vi "Read CSV.vi"(8 "error in (no error)":errorcluster caption="Error In", 10 "Source":string, 11 "Data Path":path=path "D:/NBT/01-Project/02-Processing/NBT-TestPlatform V2/NBT-TestPlatform V2.0.2/Config/NBT/NBT_V1.0.0/Project/0001_HZKD_ST01/00_DataSource/001_PLC/01_PLC/Data.xlsx") -> (0 "error out":errorcluster caption="Error Out", 1 "Data":T1(c390), 2 "Identifier List":T2[](array[typedef]), 3 "Identifiers Out":map{string, T2}(c390), 4 "Value Out":string[][](array[string]), 5 "Identifiers":string, 6 "Identifiers Out":string[](array[string]), 7 "Title":string[](array[string]))   [LabVIEW 2020]
uses:
  Global/Data Global/SDQ Data Type.ctl
  <vilib>/Utility/file.llb/Read Delimited Spreadsheet (string).vi
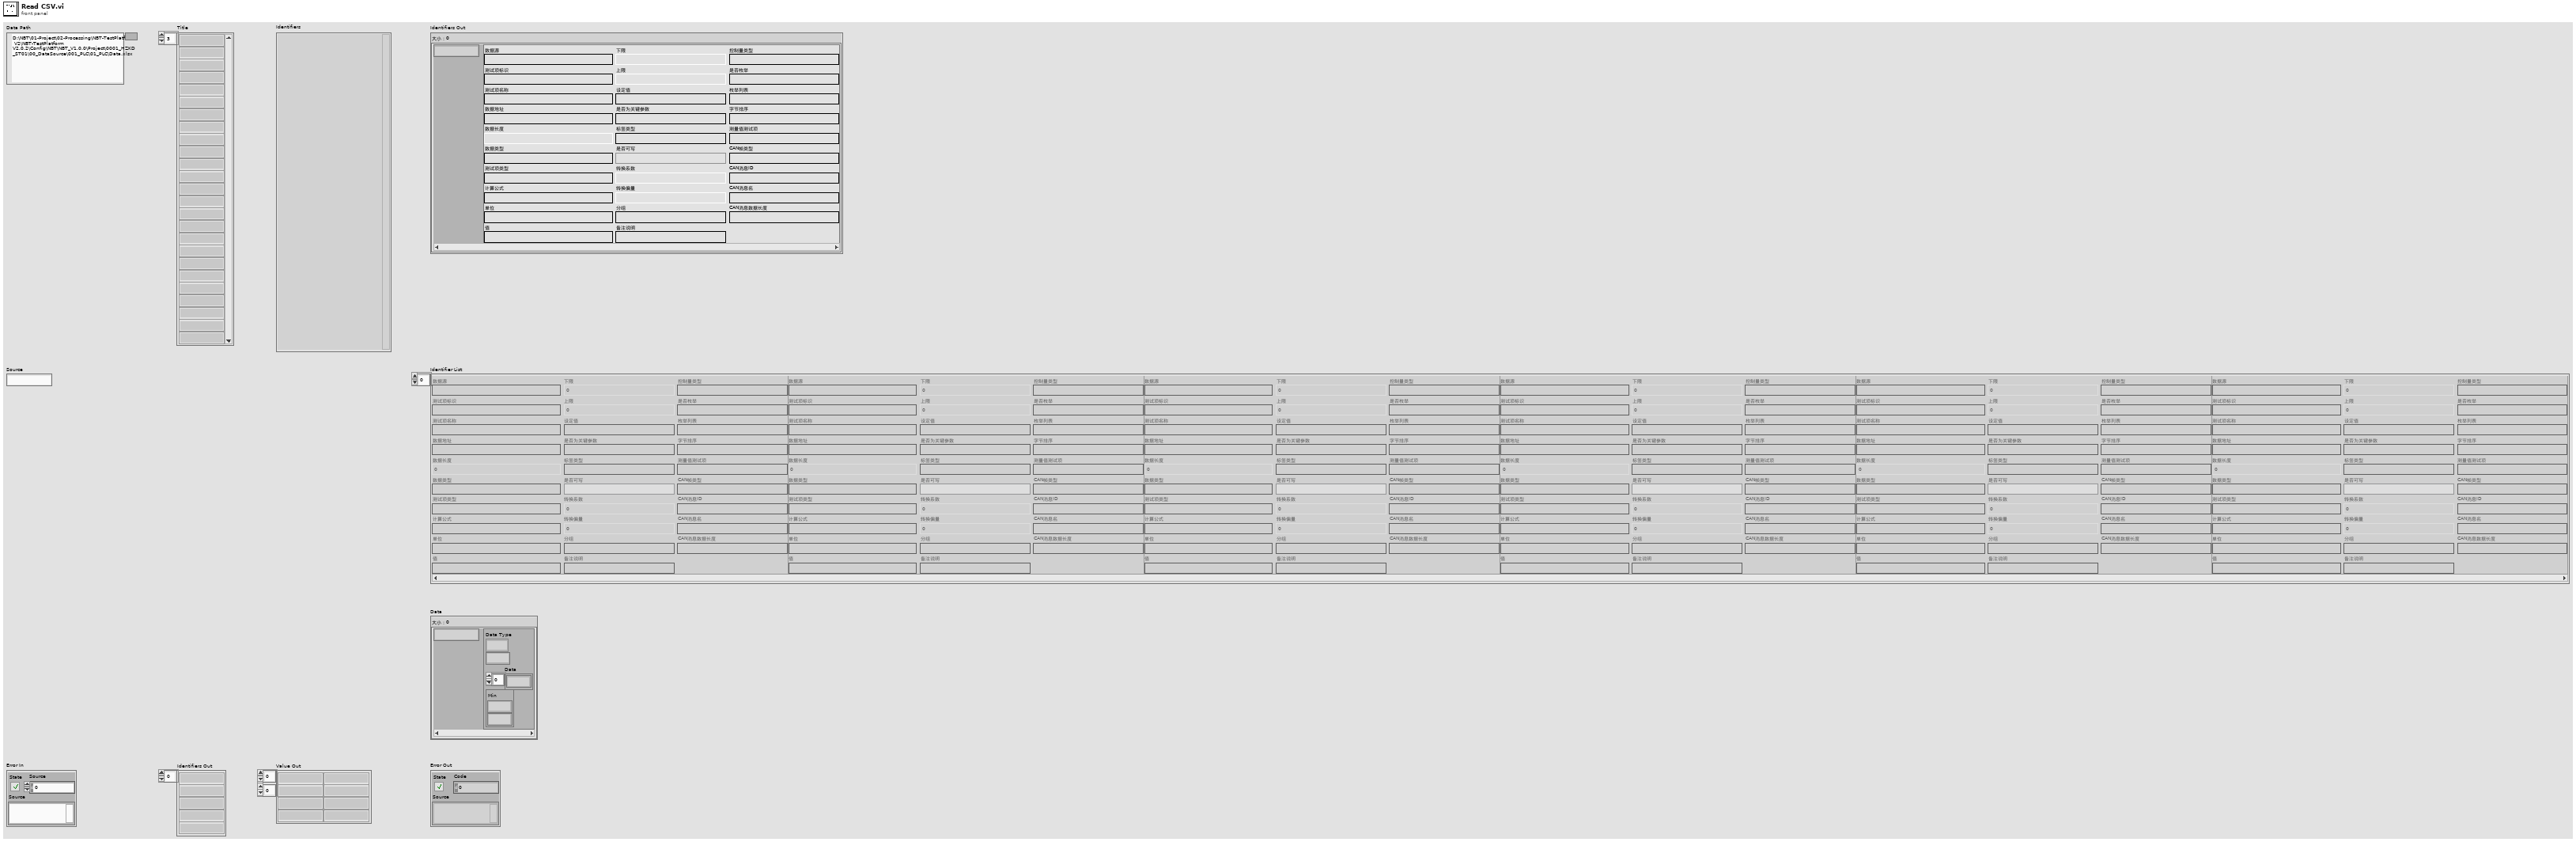
[diagram p1: front panel]
types:
  T1 = map{string, cluster{"Data Type":enum16{"I", "Q", "M", "D", "Count", "Timer"}, u16, "Data":u8[], cluster{"Min":u16, u16}}}
  T2 = typedef "SDQ Data Type.ctl" = cluster{"CAN Length":string, "CAN Name":string, "CAN ID":string, "CAN Type":string, "Test Item":string, "Byte Order":string, "Instruction":string, "Control Type":string, "Group":string, "Offset":dbl, "Coefficient":dbl, "Write Enable":bool, "Lable Type":string, "Key?":string, "Set Value":string, "Upper":dbl, "Lower":dbl, "Unit":string, "Formula":string, "Test Item Type":string, "Length":i32, "Address":string, "Name":string, "Identifier":string, "Data Type":string, "Enumerate?":string, "Enumerate List":string, "Data":string, "Source":string}
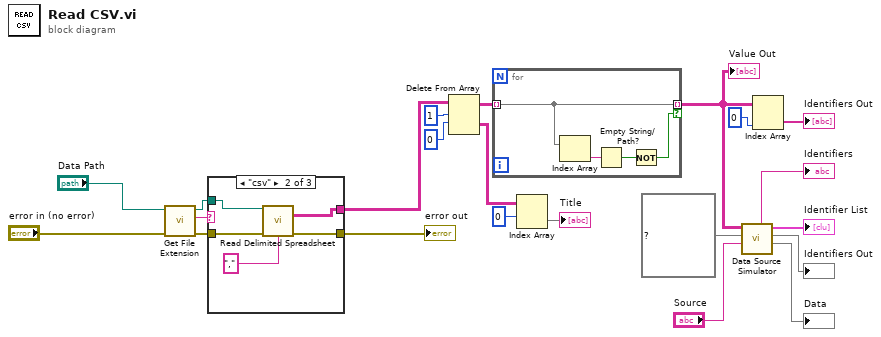
[diagram p0: block diagram]
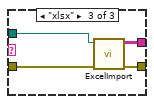
[diagram p3: hidden frame]
diagram:
  n1 = call <vilib>:"Get File Extension.vi"("error in (no error)"="error in (no error)", "file"="Data Path") -> ("error out"=w2:errorcluster, "lowercase file extension"=w1:string, "dup file"=w4:path)  [unwired: 5 in, 2 out]
  n2 = case shown="\"csv\"" w1 {
    tunnel: [_ w27 w31] -> w22
    tunnel: [w23 w26 w29] -> w19
    tunnel: w4 -> [_ w25 w32]
    tunnel: w2 -> [w23 w24 w30]
    frame Default {
    }
    frame "csv" {
      n3 = call-poly <vilib>:"Read Delimited Spreadsheet.vi"("file path (dialog if empty)"=w25, "error in (no error)"=w24, "delimiter (\\t)"="," ("delimiter (\\t)")) -> ("all rows"=w27:string[][], "error out"=w26:errorcluster)  [unwired: 7 in, 4 out]
    }
    frame "xlsx" {
      n4 = call "ExcelImport.vi"("错误输入（无错误）"=w30, "路径"=w32) -> ("错误输出"=w29:errorcluster, "All"=w31:string[][])  [unwired: 6 in, 2 out]
    }
  }
  "error out" <- w19
  n5 = Delete From Array(array=w22, length=1 ("长度"), index (row)=0 ("索引 (行)")) -> (deleted portion=w12:string[][], array with subset deleted=w15:string[][])  [unwired: 1 in]
  n6 = for {
    tunnel: [w33] -> w8 mode=indexing if=w35
    tunnel: w15 -> [w33] mode=indexing
    n7 = Index Array(array=w33) -> (element=w34:string)  [unwired: 1 in]
    n8 = Empty String/Path?(string/path=w34) -> (empty?=w36:bool)
    n9 = Not(x=w36) -> (.not. x?=w35:bool)
  }
  "Value Out" <- w8
  n10 = Index Array(array=w12, index (row)=0 ("索引 (行)")) -> (element=→"Title":string[])  [unwired: 1 in]
  n11 = call "Data Source Simulator.vi"("Source"="Source", "Identifiers In"=map{string, T2} {}, "data"=w8) -> ("Data"=→"Data":T1, "Identifiers Out"=→"Identifiers Out":map{string, T2}, "Identifier List"=→"Identifier List":T2[], "Identifiers"=→"Identifiers":string)  [unwired: 4 in, 1 out]
  n12 = Index Array(array=w8, index (col)=0 ("禁用的索引 (列)")) -> (element=→"Identifiers Out":string[])  [unwired: 1 in]
